vi "Write ITX (2D).vi"(0 "Commands":string, 5 "filename":path, 7 "Notes":string, 10 "2D Array name":string, 11 "2D Array":dbl[][](array[numeric])) -> ()   [LabVIEW 2016, in "Data.ITX.lvclass"]
uses:
  Data.ITX.lvclass
  Data/Data.lvclass
panel:
  out "String":string
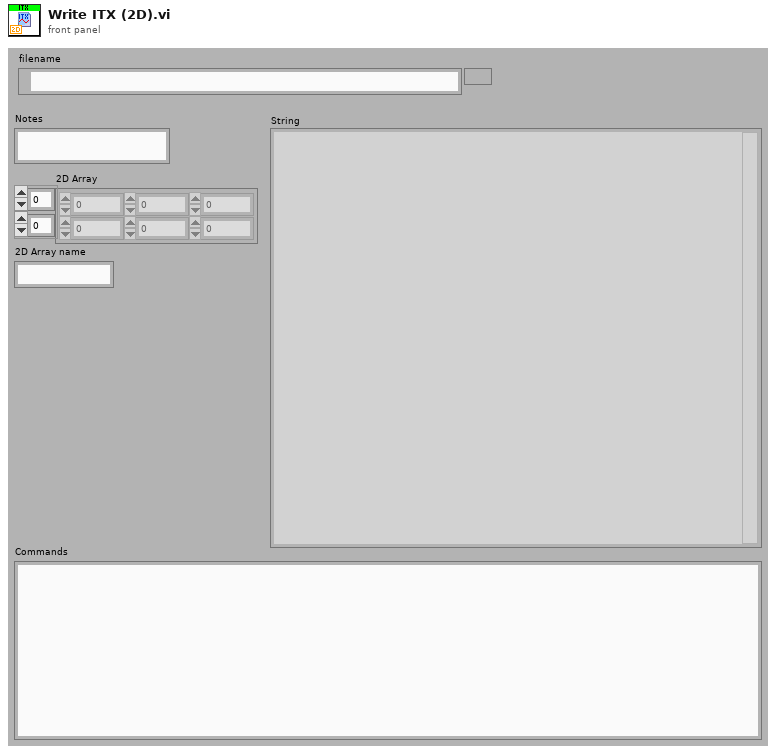
[diagram p1: front panel]
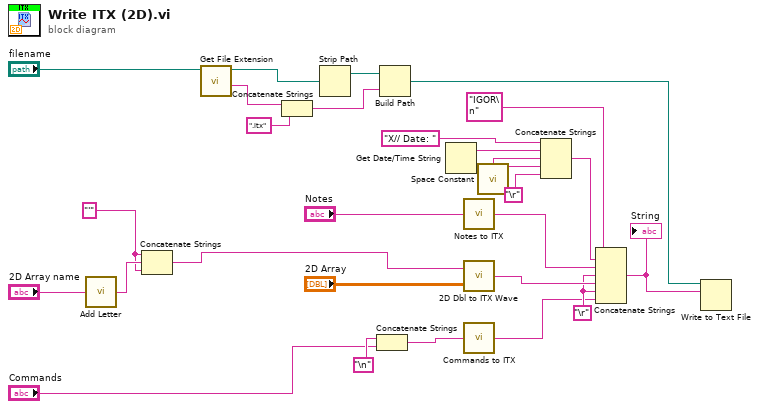
[diagram p0: block diagram]
diagram:
  w1 = "'" ("string")
  w19 = "\r"
  n1 = call "Add Letter.vi"("String"="2D Array name") -> ("output string"=w2:string)
  n2 = Concatenate Strings(w1, w2, w1) -> (w3:string)
  n3 = call <vilib>:"Get File Extension.vi"("file"="filename") -> ("filename without extension"=w15:string, "dup file"=w10:path)  [unwired: 1 in, 8 out]
  n4 = Concatenate Strings(w15, ".itx") -> (w8:string)
  n5 = Strip Path(path=w10) -> (stripped path=w9:path)  [unwired: 1 out]
  n6 = Concatenate Strings("\n", "Commands") -> (w12:string)
  n7 = Build Path(base path=w9, name or relative path=w8) -> (appended path=w11:path)
  n8 = Get Date/Time String() -> (date string=w27:string, time string=w28:string)  [unwired: 3 out]
  n9 = call "Notes to ITX.vi"("Notes"="Notes") -> ("ITX Notes"=w20:string)
  n10 = call "2D Dbl to ITX Wave.vi"("2D Array"="2D Array", "Wavename"=w3) -> ("ITX Wave"=w21:string)
  n11 = call "Commands to ITX.vi"("Commands"=w12) -> ("ITX Commands"=w4:string)
  n12 = call <vilib>:"Space Constant.vi"() -> ("String"=w17:string)
  n13 = Concatenate Strings("X// Date: " ("format string"), w27, w17, w28, "\r") -> (w26:string)
  n14 = Concatenate Strings("IGOR\n", w26, w20, w19, w21, w19, w4) -> (w18:string)
  "String" <- w18
  n15 = Write to Text File(file (use dialog)=w11, text=w18) -> ()  [unwired: 1 in, 4 out]
